vi "Last5lines (SubVI).vi"(11 "File Path Control":path) -> (1 "String Data":string[](array[string]), 2 "Last 5 Lines in\nreverse":string[](array[string]), 3 "Output":string, 4 "Number of Lines in Text File":dbl)   [LabVIEW 2013]
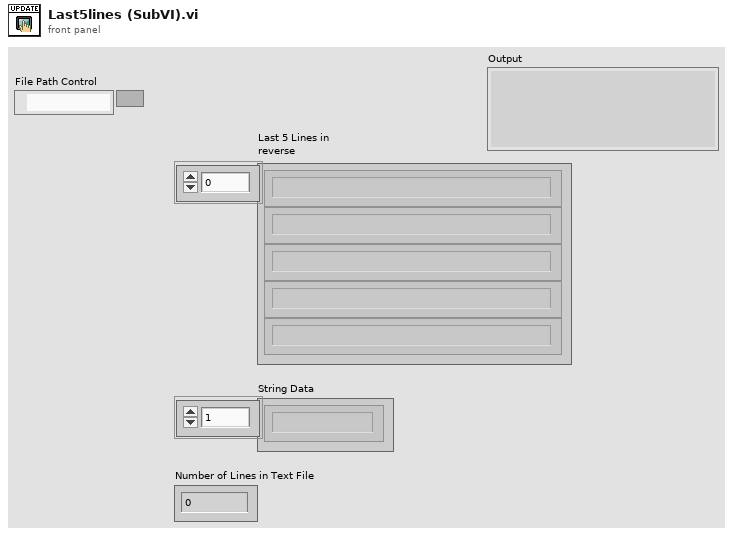
[diagram p1: front panel]
types:
  T1 = cluster{"[0]":string, "[1]":string, "[2]":string, "[3]":string, "[4]":string, "[5]":string, "[6]":string, "[7]":string, "[8]":string}
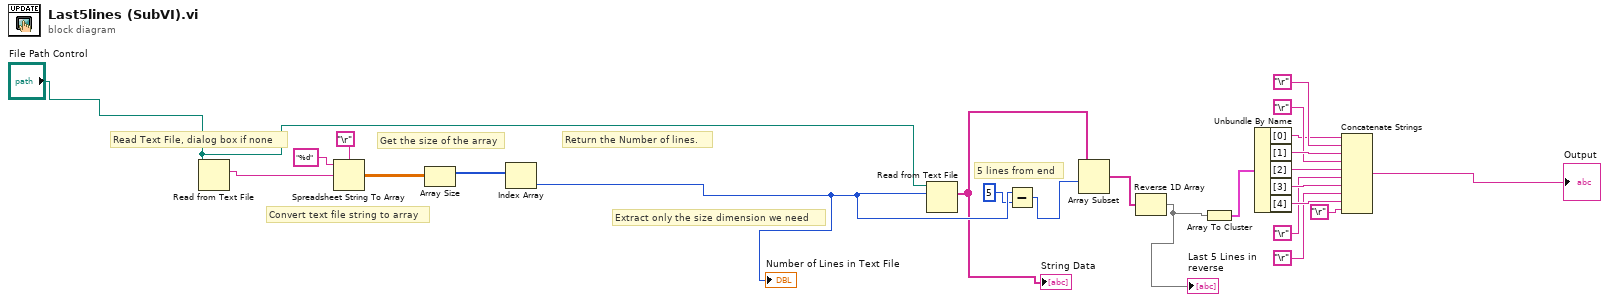
[diagram p0: block diagram]
diagram:
  # "5 lines from end"
  # "Convert text file string to array"
  # "Return the Number of lines."
  # "Extract only the size dimension we need"
  # "Get the size of the array"
  # "Read Text File, dialog box if none"
  n1 = Read from Text File(file (use dialog)="File Path Control") -> (text=w5:string)  [unwired: 1 in, 5 out]
  n2 = Spreadsheet String To Array(delimiter (Tab)="\r", format string="%d", spreadsheet string=w5) -> (array=w3:dbl[][])  [unwired: 1 out]
  n3 = Array Size(array=w3) -> (size(s)=w4:i32[])
  n4 = Index Array(array=w4) -> (element=w9:i32)  [unwired: 1 in]
  "Number of Lines in Text File" <- w9
  n5 = Read from Text File(file (use dialog)="File Path Control", count=w9) -> (text=w7:string[])  [unwired: 1 in, 4 out]
  "String Data" <- w7
  n6 = Subtract(x=w9, y=5 ("x")) -> (x-y=w10:i32)
  n7 = Array Subset(array=w7, index=w10) -> (w11:string[])  [unwired: 1 in]
  n8 = Reverse 1D Array(array=w11) -> (reversed array=w12:string[])
  "Last 5 Lines in\nreverse" <- w12
  n9 = Array To Cluster(array=w12) -> (cluster=w13:T1)
  n10 = Unbundle By Name(w13) -> ("[0]"=w14:string, "[1]"=w18:string, "[2]"=w19:string, "[3]"=w22:string, "[4]"=w23:string)
  n11 = Concatenate Strings(w14, "\r", w18, "\r", w19, "\r", w22, "\r", w23, "\r") -> (→"Output":string)
